vi "ToggleCommand.vi"(7 "Item Ref in":T1 format="%.0x", 8 "error in (no error)":errorcluster, 9 "On Segmentation":bool, 10 "Property Name":string, 11 "String in":refnum<vi>) -> (0 "error out":errorcluster)   [LabVIEW 2024, in "Embedded TDMS Logger System Explorer.lvlib"]
uses:
  Embedded TDMS Logger System Explorer.lvlib
  <vilib>/NI VeriStand/Custom Device API/Custom Device API.lvlib
  <vilib>/NI VeriStand/Custom Device API/Set Item Property (String).vi
  <vilib>/NI VeriStand/Custom Device API/Custom Device Item Ref.ctl
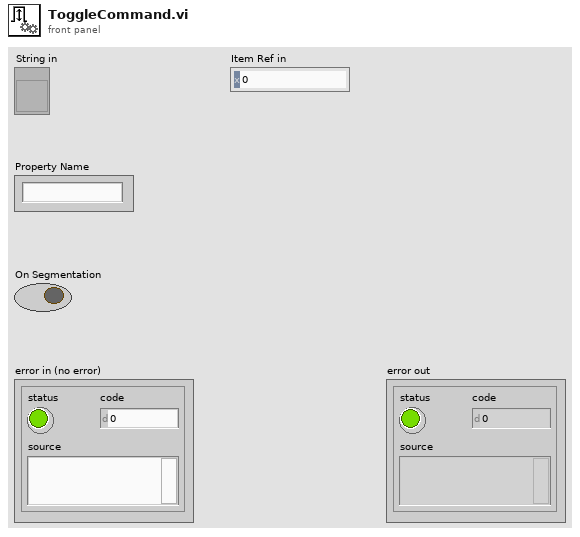
[diagram p1: front panel]
types:
  T1 = typedef "Custom Device API.lvlib/Custom Device Item Ref.ctl" = u64
  T2 = enum8{"Enabled", "Disabled", "Disabled and Grayed Out"}
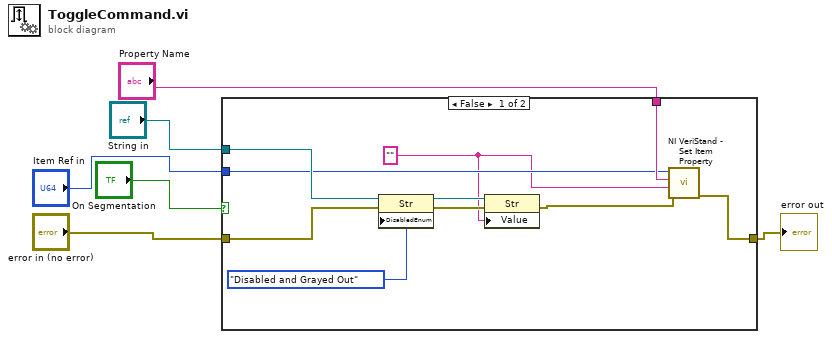
[diagram p0: block diagram]
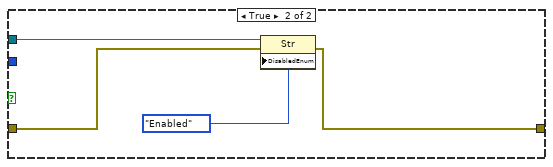
[diagram p2: hidden frame]
diagram:
  n1 = case shown="False" "On Segmentation" {
    tunnel: "String in" -> [w14 w20]
    tunnel: "error in (no error)" -> [w15 w18]
    tunnel: [w13 w17] -> w4
    tunnel: "Property Name" -> [w12 _]
    tunnel: "Item Ref in" -> [w11 _]
    frame False {
      w7 = "" ("Value")
      n2 = property class="Str"(reference=w14, error in=w15, "DisabledEnum"=T2."Disabled and Grayed Out" ("Disabled")) -> (reference out=w9:refnum<vi>, error out=w10:errorcluster)
      n3 = property class="Str"(reference=w9, error in=w10, "Value"=w7) -> (error out=w8:errorcluster)  [unwired: 1 out]
      n4 = call-poly <vilib>:"NI VeriStand - Set Item Property.vi"("error in (no error)"=w8, "Value"=w7, "Property Name"=w12, "Item Ref in"=w11) -> ("error out"=w13:errorcluster)  [unwired: 5 in, 2 out]
    }
    frame True {
      n5 = property class="Str"(reference=w20, error in=w18, "DisabledEnum"=T2."Enabled" ("Disabled")) -> (error out=w17:errorcluster)  [unwired: 1 out]
    }
  }
  "error out" <- w4
